vi "Animation Done Callback VI Type.vi"(11 "Owner":refnum<class>) -> ()   [LabVIEW 2020, in "PicoG-Processor.lvlib"]
uses:
  PicoG-Processor.lvlib
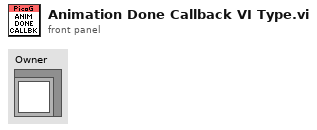
[diagram p1: front panel]
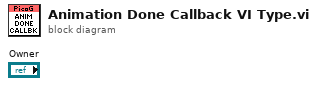
[diagram p0: block diagram]
diagram:
